vi "RH_DCPower_ConfigureSequence.vi"(7 "DCPower_SequenceParameters":T1 {"DeltaVoltage" format="%.6p"; "DeltaTime" format="%.6p"; "Voltage Stop" format="%.6p"; "Aperture_time" format="%.6p"; "Current_range" format="%.6p"; "Current" format="%.6p"; "Voltage_range" format="%.6p"; "Voltage Start" format="%.6p"}, 8 "error in (no error)":errorcluster, 9 "Peak duration (s)":dbl, 10 "channel name":string, 11 "DCPower Session In":refnum<k15>) -> (0 "error out":errorcluster, 1 "num points":i32, 3 "DCPower Session Out":refnum<k15>)   [LabVIEW 2023, in "ResourceHandling.lvlib"]
doc: "Configure the SMU in Sequence Mode setting also the Aperture Time"
uses:
  ResourceHandling.lvlib
  TypeDefs/RH_DCPower_SequenceParameters.ctl
  <instrlib>/niDCPower/nidcpower.llb/niDCPower Output Function.ctl
  <instrlib>/niDCPower/nidcpower.llb/niDCPower Source Mode.ctl
  <instrlib>/niDCPower/nidcpower.llb/niDCPower Aperture Time Units.ctl
  <vilib>/Analysis/1siggen.llb/Ramp Pattern by Delta.vi
  <vilib>/Analysis/NI_AALBase.lvlib
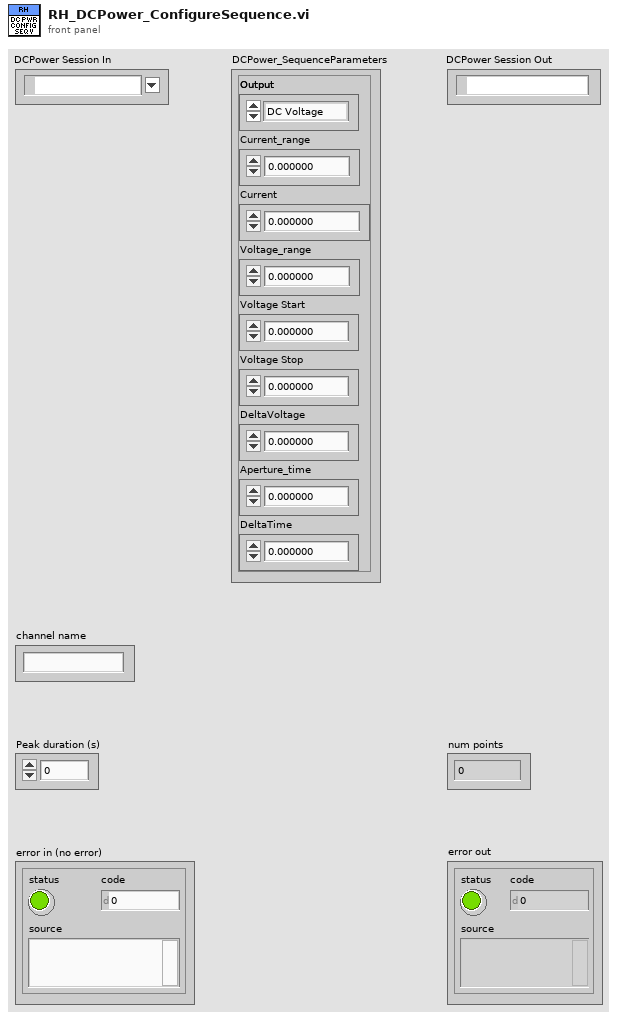
[diagram p1: front panel]
types:
  T1 = typedef "ResourceHandling.lvlib/RH_DCPower_SequenceParameters.ctl" = cluster{"Output":enum16{"DC Voltage", "DC Current"}, "Current_range":dbl, "Current":dbl, "Voltage_range":dbl, "Voltage Start":dbl, "Voltage Stop":dbl, "DeltaVoltage":dbl, "Aperture_time":dbl, "DeltaTime":dbl}
  T2 = typedef "niDCPower Source Mode.ctl" = i32
  T3 = typedef "niDCPower Output Function.ctl" = i32
  T4 = typedef "niDCPower Aperture Time Units.ctl" = i32
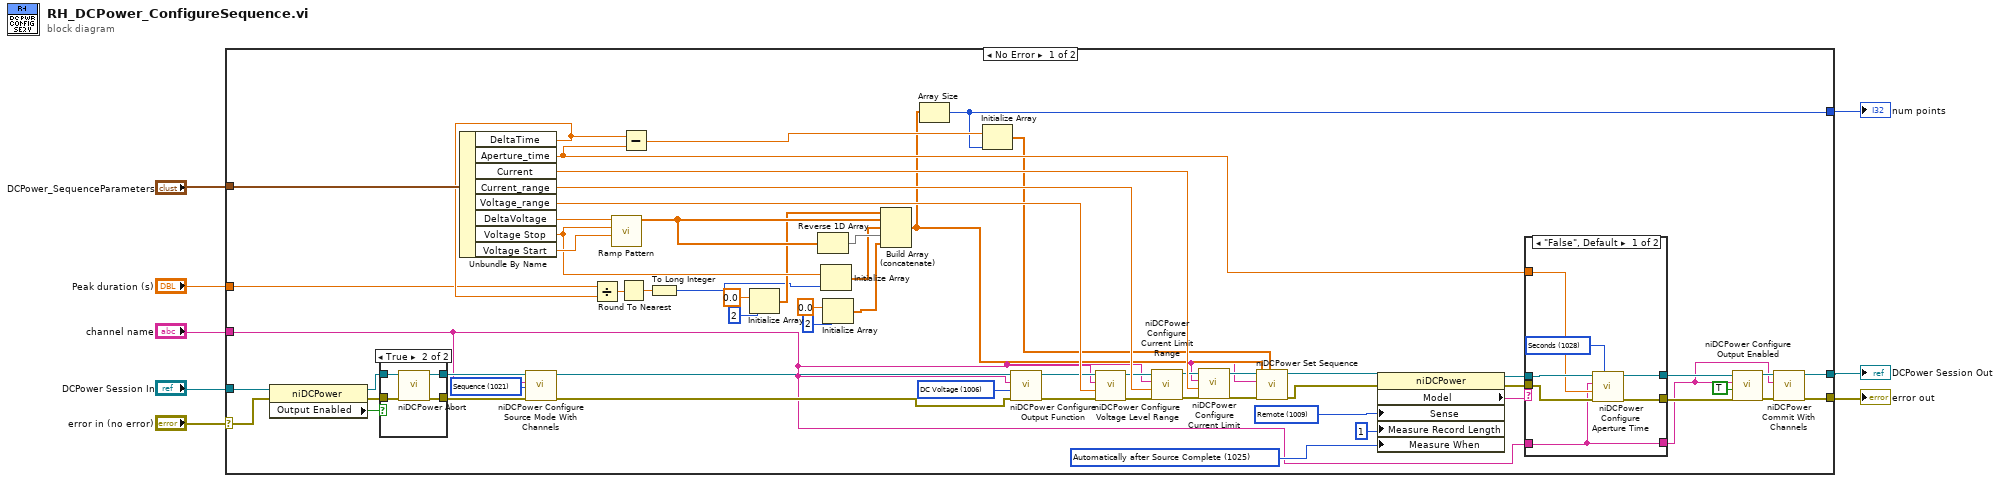
[diagram p0: block diagram]
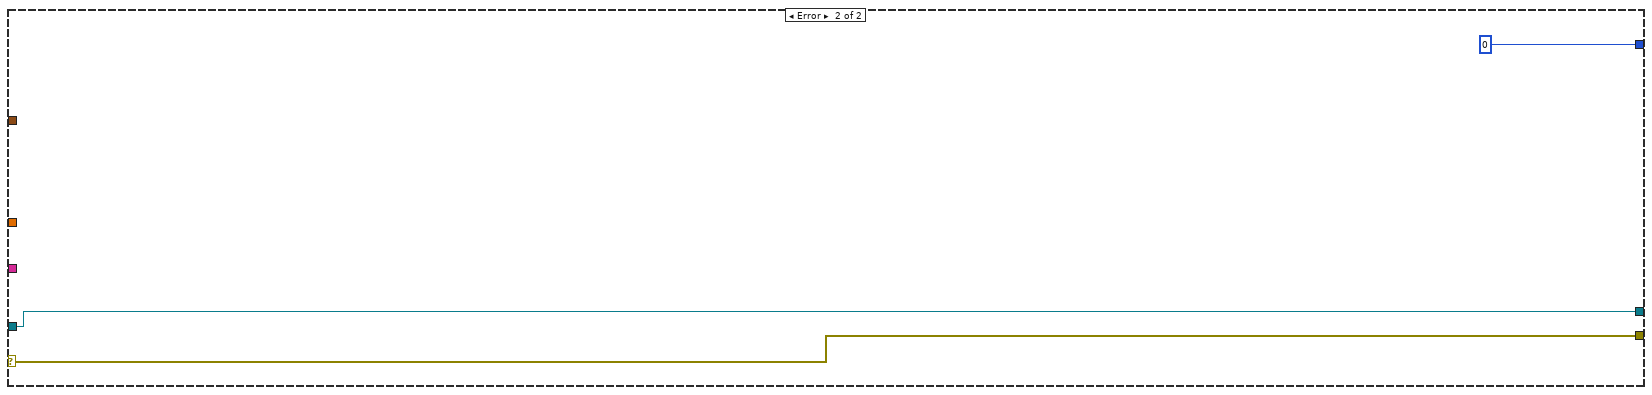
[diagram p4: hidden frame]
diagram:
  n1 = case shown="No Error" "error in (no error)" {
    selector: "error in (no error)" -> [w53 w89]
    tunnel: "DCPower Session In" -> [w56 w88]
    tunnel: [w55 w88] -> w1
    tunnel: [w54 w89] -> w8
    tunnel: "channel name" -> [w10 _]
    tunnel: "DCPower_SequenceParameters" -> [w44 _]
    tunnel: "Peak duration (s)" -> [w24 _]
    tunnel: [w20 0] -> w3
    frame No Error {
      w12 = 1025 items=["Automatically after Source Complete"=1025, "On Demand"=1026, "On Measure Trigger"=1027] ("Measurement:Advanced:Measure When")
      w15 = 1009 items=["Local"=1008, "Remote"=1009] ("Measurement:Sense")
      w45 = T2 1021 items=["Single Point"=1020, "Sequence"=1021] ("source mode")
      w52 = T3 1006 items=["DC Voltage"=1006, "DC Current"=1007, "Pulse Voltage"=1049, "Pulse Current"=1050] ("output function")
      n2 = property class="niDCPower"(reference=w56, error in=w53) -> (reference out=w68:refnum<k15>, error out=w69:errorcluster, "Output Enabled"=w67:bool)
      n3 = case shown="True" w67 {
        tunnel: w68 -> [w82 w86]
        tunnel: w69 -> [w81 w85]
        tunnel: [w82 w84] -> w46
        tunnel: [w81 w83] -> w47
        frame False {
        }
        frame True {
          n4 = call <instrlib>:"niDCPower Abort.vi"("error in (no error)"=w85, "instrument handle"=w86) -> ("error out"=w83:errorcluster, "instrument handle out"=w84:refnum<k15>)  [unwired: 8 in]
        }
      }
      n5 = Unbundle By Name(w44) -> ("DeltaTime"=w25:dbl, "Aperture_time"=w43:dbl, "Current"=w62:dbl, "Current_range"=w63:dbl, "Voltage_range"=w64:dbl, "DeltaVoltage"=w40:dbl, "Voltage Stop"=w35:dbl, "Voltage Start"=w39:dbl)
      n6 = call <instrlib>:"niDCPower Configure Source Mode With Channels.vi"("error in (no error)"=w47, "source mode"=w45, "channel name"=w10, "instrument handle"=w46) -> ("error out"=w14:errorcluster, "instrument handle out"=w13:refnum<k15>)  [unwired: 6 in]
      n7 = Divide(x=w24, y=w25) -> (x/y=w23:dbl)
      n8 = call-poly <vilib>:"Ramp Pattern.vi"("start"=w39, "end"=w35, "delta"=w40) -> ("Ramp Pattern"=w37:dbl[])  [unwired: 6 in, 2 out]
      n9 = Round To Nearest(number=w23) -> (nearest integer value=w22:dbl)
      n10 = Subtract(x=w25, y=w43) -> (x-y=w38:dbl)
      n11 = To Long Integer(number=w22) -> (32bit integer=w21:i32)
      n12 = Initialize Array(0.0 ("element"), 2 ("dimension size")) -> (w29:dbl[])
      n13 = Reverse 1D Array(array=w37) -> (reversed array=w36:dbl[])
      n14 = Initialize Array(w35, w21) -> (w34:dbl[])
      n15 = Initialize Array(0.0 ("element"), 2 ("dimension size")) -> (w32:dbl[])
      n16 = Build Array (concatenate)(w29, w37, w34, w36, w32) -> (w28:dbl[])
      n17 = Array Size(array=w28) -> (size(s)=w20:i32)
      n18 = Initialize Array(w38, w20) -> (w27:dbl[])
      n19 = call <instrlib>:"niDCPower Configure Output Function.vi"("error in (no error)"=w14, "output function"=w52, "channel name"=w10, "instrument handle"=w13) -> ("error out"=w41:errorcluster, "instrument handle out"=w42:refnum<k15>)  [unwired: 6 in]
      n20 = call <instrlib>:"niDCPower Configure Voltage Level Range.vi"("error in (no error)"=w41, "voltage level range"=w64, "channel name"=w10, "instrument handle"=w42) -> ("error out"=w51:errorcluster, "instrument handle out"=w50:refnum<k15>)  [unwired: 6 in]
      n21 = call <instrlib>:"niDCPower Configure Current Limit Range.vi"("error in (no error)"=w51, "current limit range"=w63, "channel name"=w10, "instrument handle"=w50) -> ("error out"=w49:errorcluster, "instrument handle out"=w48:refnum<k15>)  [unwired: 6 in]
      n22 = call <instrlib>:"niDCPower Configure Current Limit.vi"("error in (no error)"=w49, "current limit"=w62, "channel name"=w10, "instrument handle"=w48) -> ("error out"=w19:errorcluster, "instrument handle out"=w16:refnum<k15>)  [unwired: 6 in]
      n23 = call <instrlib>:"niDCPower Set Sequence.vi"("source delays"=w27, "error in (no error)"=w19, "values"=w28, "channel name"=w10, "instrument handle"=w16) -> ("error out"=w18:errorcluster, "instrument handle out"=w17:refnum<k15>)  [unwired: 5 in]
      n24 = property class="niDCPower"(reference=w17, error in=w18, "Sense"=w15, "Measure Record Length"=1 ("Measurement:Measure Record Length"), "Measure When"=w12) -> (reference out=w60:refnum<k15>, error out=w59:errorcluster, "Model"=w61:string)
      n25 = case shown="\"False\", Default" w61 {
        tunnel: w60 -> [w77 w80]
        tunnel: w59 -> [w76 w79]
        tunnel: [w75 w79] -> w58
        tunnel: [w74 w80] -> w57
        tunnel: w43 -> [w73 _]
        tunnel: w10 -> [w71 w78]
        tunnel: [w71 w78] -> w9
        frame "False", Default {
          w72 = T4 1028 items=["Seconds"=1028, "Powerline Cycles"=1029] ("aperture time units")
          n26 = call <instrlib>:"niDCPower Configure Aperture Time.vi"("aperture time units"=w72, "error in (no error)"=w76, "aperture time"=w73, "channel name"=w71, "instrument handle"=w77) -> ("error out"=w75:errorcluster, "instrument handle out"=w74:refnum<k15>)  [unwired: 5 in]
        }
        frame "NI PXI-4110" {
        }
      }
      n27 = call <instrlib>:"niDCPower Configure Output Enabled.vi"("error in (no error)"=w58, "output enabled"=TRUE, "channel name"=w9, "instrument handle"=w57) -> ("error out"=w66:errorcluster, "instrument handle out"=w65:refnum<k15>)  [unwired: 6 in]
      n28 = call <instrlib>:"niDCPower Commit With Channels.vi"("error in (no error)"=w66, "channel name"=w9, "instrument handle"=w65) -> ("error out"=w54:errorcluster, "instrument handle out"=w55:refnum<k15>)  [unwired: 7 in]
    }
    frame Error {
    }
  }
  "error out" <- w8
  "num points" <- w3
  "DCPower Session Out" <- w1
